vi "FTW-TestStep-Wait-Core_Initialize.vi"(0 "Initialization Sequence":string, 5 "FTW Actor Instance Configuration":string, 11 "error in (no error)":errorcluster) -> (4 "FTW-TestStep-Wait-Core Out":refnum<class "FTW-TestStep-Wait-Core.lvclass">, 6 "Event Refnums":T1, 10 "Wait Time":dbl, 15 "error out":errorcluster)   [LabVIEW 2018, in "FTW-TestStep-Wait-Core.lvclass"]
uses:
  FTW-TestStep-Wait-Core.lvclass
  C:/Jobs/Featherweight/featherweight-2018/source/actor/TestStepBase/FTW-TestStep-Base.lvclass
  source/actor/Message/Request/FTW-Message-IncomingRequest.lvclass
  source/actor/Message/Base/FTW-Message.lvclass
  3f365fc9-e691-4620-b02e-8c1061e90582.vi
  source/JSON/core/FTW-JSON-Core-EncodingFlags.vi
  source/Reflection/FTW-Reflection-Type.vi
  source/JSON/FTW-JSON-Parse.vi
  source/container/FTW-Container-GetFlattenedValue.vi
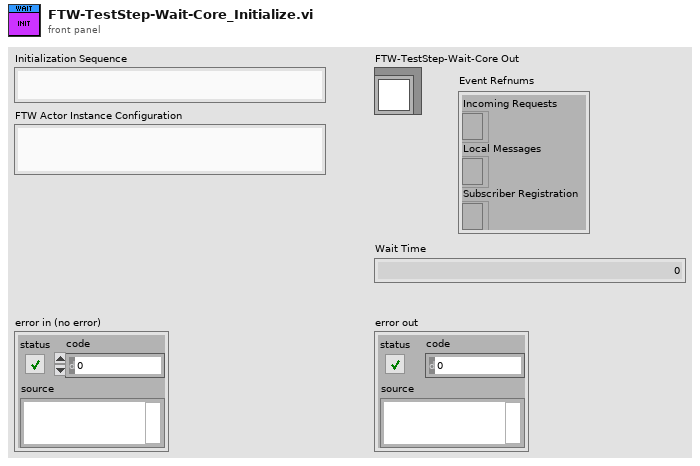
[diagram p1: front panel]
types:
  T1 = cluster{"Incoming Requests":refnum<event-registration>, "Local Messages":refnum<event-registration>, "Subscriber Registration":refnum<event-registration>}
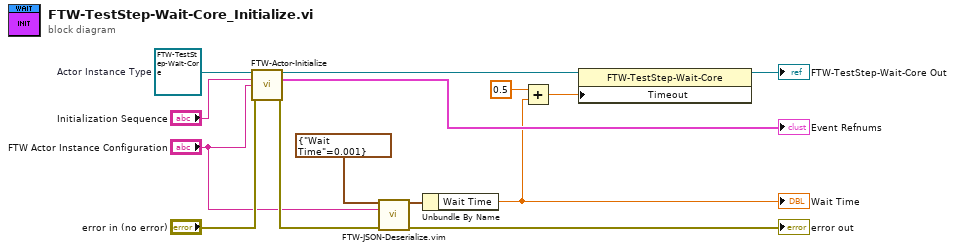
[diagram p0: block diagram]
diagram:
  w14 = refnum<class "FTW-TestStep-Wait-Core.lvclass"> refnum  # Actor Instance Type
  n1 = call-dynamic "FTW-Actor-Initialize.vi"("FTW Actor Instance Type"=w14, "Initialization Job Sequence"="Initialization Sequence", "Actor Instance Configuration"="FTW Actor Instance Configuration", "error in"="error in (no error)") -> ("FTW Actor Instance"=w10:refnum<class "FTW-TestStep-Wait-Core.lvclass">, "Event Refnums"=→"Event Refnums":T1, "error out"=w8:errorcluster)  [unwired: 9 in]
  n2 = call "FTW-JSON-Deserialize.vim"("Type In"=cluster{"Wait Time":dbl} {"Wait Time"=0.001} ("Type and Defaults"), "JSON String"="FTW Actor Instance Configuration", "error in"=w8) -> ("Type Out"=w11:cluster{"Wait Time":dbl}, "error out"=→"error out":errorcluster)  [unwired: 11 in]
  n3 = Unbundle By Name(w11) -> ("Wait Time"=w3:dbl)
  "Wait Time" <- w3
  n4 = Add(x=0.5, y=w3) -> (x+y=w1:dbl)
  n5 = property class="FTW-TestStep-Wait-Core"(reference=w10, "Timeout"=w1) -> (reference out=→"FTW-TestStep-Wait-Core Out":refnum<class "FTW-TestStep-Wait-Core.lvclass">)  [unwired: 1 in, 1 out]
